vi "junk.vi"() -> ()   [LabVIEW 2013]
panel:
  out "Numeric":i32
  in  "timeout ms (-1 never timeout)":i32
  in  "front panel (this VI's panel)":refnum<vi>
  in  "do not wait! (False)":bool
  out "Column":i32
  out "Row":i32
  out "Item Names":string[][](array[string])
  out "element":string
  out "Multicolumn Listbox 2":i32(listbox)
  in  "Multicolumn Listbox":i32(listbox)
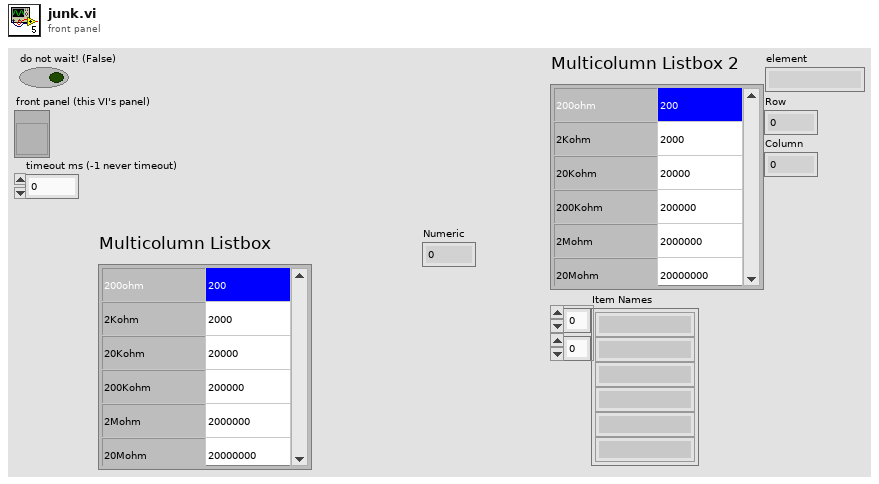
[diagram p1: front panel]
types:
  T1 = typedef "LVRowAndColumnTypeDef.ctl" = cluster{"Row":i32, "Column":i32}
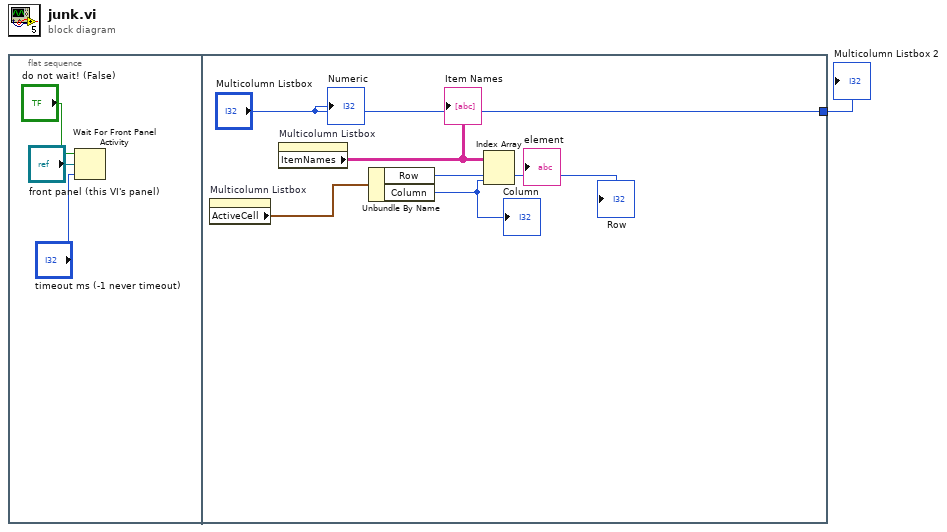
[diagram p0: block diagram]
diagram:
  n1 = flat-sequence {
    tunnel: ["Multicolumn Listbox"] -> w1
    frame #0 {
      n2 = Wait For Front Panel Activity(1:"timeout ms (-1 never timeout)", 2:"front panel (this VI's panel)", 3:"do not wait! (False)") -> ()  [unwired: 1 out]
    }
    frame #1 {
      n3 = property on="Multicolumn Listbox" class="MCListbox (strict)"() -> ("ActiveCell"=w9:T1)  [unwired: 2 in, 2 out]
      n4 = property on="Multicolumn Listbox" class="MCListbox (strict)"() -> ("ItemNames"=w10:string[][])  [unwired: 2 in, 2 out]
      "Item Names" <- w10
      n5 = Unbundle By Name(w9) -> ("Row"=w8:i32, "Column"=w7:i32)
      "Row" <- w8
      "Column" <- w7
      n6 = Index Array(array=w10, index (row)=w8, index (col)=w7) -> (element=→"element":string)
      "Numeric" <- "Multicolumn Listbox"
    }
  }
  "Multicolumn Listbox 2" <- w1
